vi "draw.vi"(8 "error in (no error)":errorcluster, 11 "fwCircle in":refnum<class "fwCircle.lvclass">) -> (0 "error out":errorcluster, 2 "Output":string, 3 "fwCircle out":refnum<class "fwCircle.lvclass">)   [LabVIEW 2017, in "fwCircle.lvclass"]
uses:
  fwCircle.lvclass
  fwCircle.lvclass/fwCircle.ctl
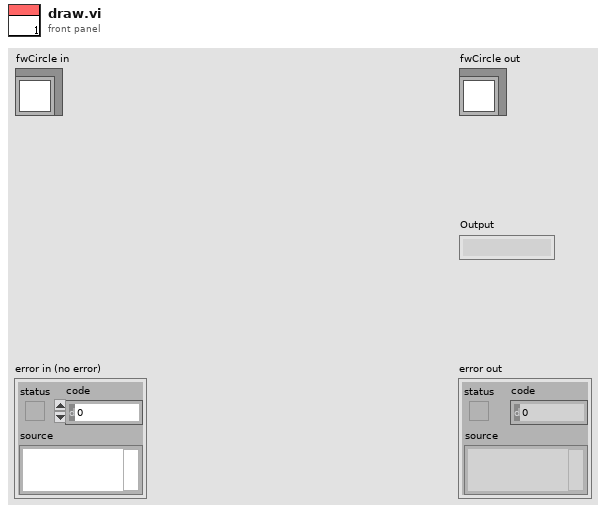
[diagram p1: front panel]
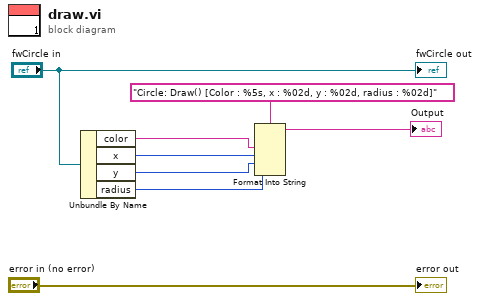
[diagram p0: block diagram]
diagram:
  n1 = Unbundle By Name("fwCircle in") -> ("color"=w5:string, "x"=w4:i32, "y"=w3:i32, "radius"=w2:i32)
  n2 = Format Into String(format string="Circle: Draw() [Color : %5s, x : %02d, y : %02d, radius : %02d]", w5, w4, w3, w2) -> (resulting string=→"Output":string)  [unwired: 2 in, 1 out]
  "error out" <- "error in (no error)"
  "fwCircle out" <- "fwCircle in"
